vi "Write File Prefix.vi"(8 "error in (no error)":errorcluster, 10 "File Prefix":string="p", 11 "File in":refnum<class "File.lvclass">) -> (0 "error out":errorcluster, 3 "File out":refnum<class "File.lvclass">)   [LabVIEW 2016, in "File.lvclass"]
uses:
  File.lvclass
  File.lvclass/File.ctl
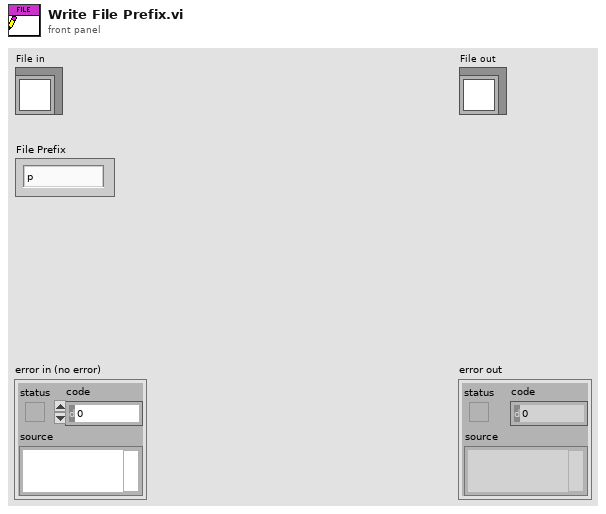
[diagram p1: front panel]
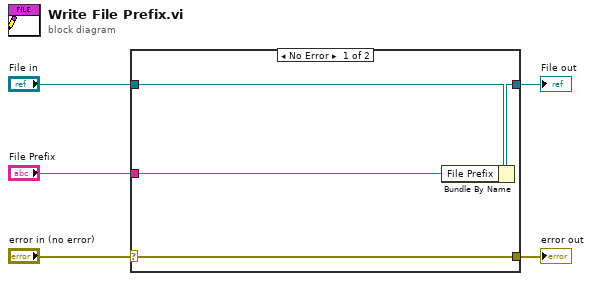
[diagram p0: block diagram]
diagram:
  n1 = case shown="No Error" "error in (no error)" {
    selector: "error in (no error)" -> [w9 w10]
    tunnel: [w9 w10] -> w4
    tunnel: [w7 w11] -> w2
    tunnel: "File in" -> [w8 w11]
    tunnel: "File Prefix" -> [w6 _]
    frame No Error {
      n2 = Bundle By Name(cluster=w8, "File Prefix"=w6) -> (w7:refnum<class "File.lvclass">)
    }
    frame Error {
    }
  }
  "error out" <- w4
  "File out" <- w2
